vi "Create Platform Application.vi"(6 "Platform Application Attributes":T1[](array[typedef]), 7 "Region":T3, 8 "error in (no error)":errorcluster, 9 "Platform":T5, 10 "Name":string, 11 "AWS Credentials":T4) -> (0 "error out":errorcluster, 3 "Platform application out":refnum<class "Platform Application.lvclass">)   [LabVIEW 2015, in "NI_AWS_SNS.lvlib" / "Platform Application.lvclass"]
uses:
  Platform Application.lvclass
  Platform.ctl
  Core/HTTP Request/AWS Credentials.ctl
  Core/HTTP Request/Region.ctl
  Application Attribute Value Pair.ctl
  Application Attribute.ctl
  Core/HTTP Request/Name Value Pair.ctl
  Core/HTTP Request/Request Options.ctl
  Core/HTTP Request/HTTP Request.lvclass/HTTP Request.ctl
  Core/ARN/ARN.lvclass/ARN.ctl
  Core/HTTP Request/Write Credentials.vi
  Core/HTTP Request/Write Region.vi
  Core/HTTP Request/Write Service.vi
  Core/HTTP Request/Write Verify Server.vi
  Core/ARN/Write ARN.vi
  Core/HTTP Request/HTTP Request.lvclass
panel:
  out "Platform application ARN":string
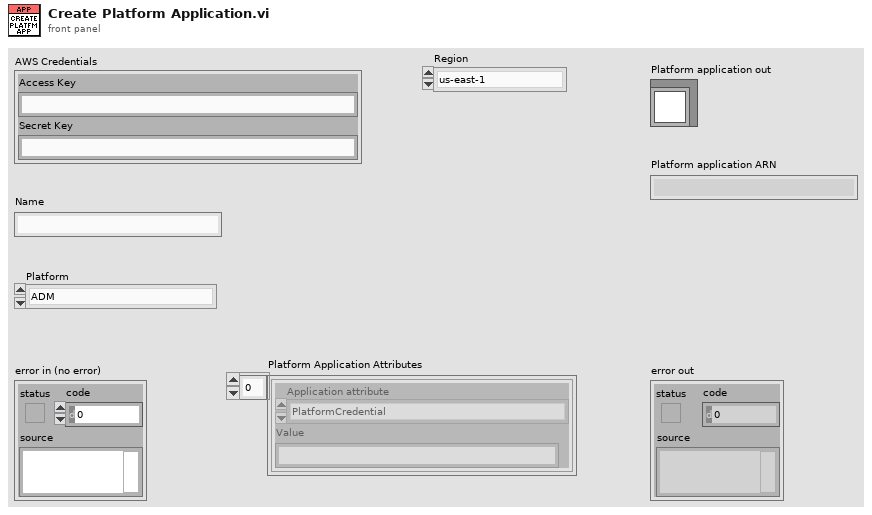
[diagram p1: front panel]
types:
  T1 = typedef "NI_AWS_SNS.lvlib/Platform Application.lvclass/Application Attribute Value Pair.ctl" = cluster{"Application attribute":T2, "Value":string}
  T2 = typedef "NI_AWS_SNS.lvlib/Platform Application.lvclass/Application Attribute.ctl" = enum16{"PlatformCredential", "PlatformPrincipal", "EventEndpointCreated", "EventEndpointDeleted", "EventEndpointUpdated", "EventDeliveryFailure", "SuccessFeedbackRoleArn", "FailureFeedbackRoleArn", "SuccessFeedbackSampleRate"}
  T3 = typedef "NI_AWS_Core.lvlib/HTTP Request.lvclass/Region.ctl" = enum16{"us-east-1", "us-east-2", "us-west-1", "us-west-2", "ap-northeast-1", "ap-northeast-2", "ap-southeast-1", "ap-southeast-2", "ca-central-1", "eu-central-1", "eu-west-1", "eu-west-2", "sa-east-1"}
  T4 = typedef "NI_AWS_Core.lvlib/HTTP Request.lvclass/AWS Credentials.ctl" = cluster{"Access Key":string, "Secret Key":string}
  T5 = typedef "NI_AWS_SNS.lvlib/Platform Application.lvclass/Platform.ctl" = enum16{"ADM", "APNS", "APNS_SANDBOX", "GCM"}
  T6 = typedef "NI_AWS_Core.lvlib/HTTP Request.lvclass/Request Options.ctl" = cluster{"request headers":T7[], "request parameters":T7[], "request body":string}
  T7 = typedef "NI_AWS_Core.lvlib/HTTP Request.lvclass/Name Value Pair.ctl" = cluster{"name":string, "value":string}
  T8 = typedef "NI_AWS_Core.lvlib/HTTP Request.lvclass/Response.ctl" = cluster{"Headers":string, "Body":string}
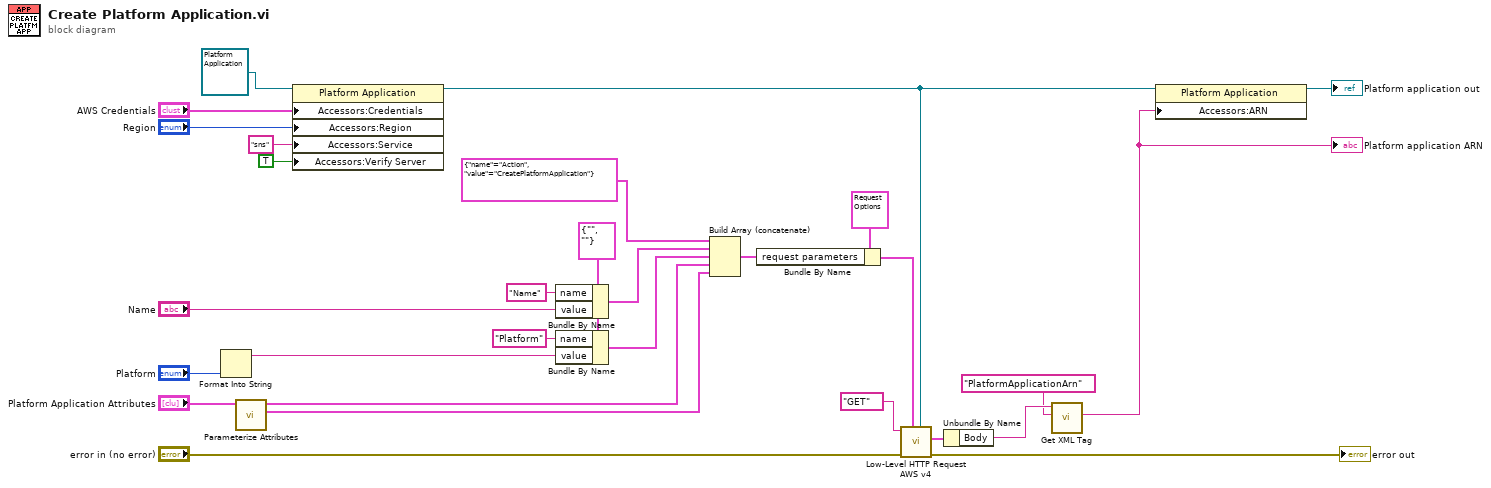
[diagram p0: block diagram]
diagram:
  w10 = T7 {"name"="", "value"=""} ("element")
  n1 = Format Into String("Platform") -> (resulting string=w7:string)  [unwired: 3 in, 1 out]
  n2 = call "Parameterize Attributes.vi"("Platform Application Attributes"="Platform Application Attributes") -> ("values"=w1:T7[], "attributes"=w2:T7[])  [unwired: 9 in]
  n3 = property class="Platform Application"(reference=refnum<class "Platform Application.lvclass"> refnum ("NI_SNS.lvclass"), "Accessors:Credentials"="AWS Credentials", "Accessors:Region"="Region", "Accessors:Service"="sns" ("Service"), "Accessors:Verify Server"=TRUE ("Verify Server")) -> (reference out=w16:refnum<class "Platform Application.lvclass">)  [unwired: 1 in, 1 out]
  n4 = Bundle By Name(cluster=w10, "name"="Name", "value"="Name") -> (w11:T7)
  n5 = Bundle By Name(cluster=w10, "name"="Platform", "value"=w7) -> (w9:T7)
  n6 = Build Array (concatenate)(T7 {"name"="Action", "value"="CreatePlatformApplication"} ("Name Value Pair"), w11, w9, w2, w1) -> (w21:T7[])
  n7 = Bundle By Name(cluster=T6 {"request headers"=[], "request parameters"=[{"name"="Action", "value"="ListQueues"}], "request body"=""} ("Request Options"), "request parameters"=w21) -> (w18:T6)
  n8 = call "Low-Level HTTP Request AWS v4.vi"("AWS Core"=w16, "Request Options"=w18, "error in (no error)"="error in (no error)", "HTTP-Verb"="GET") -> ("error out"=→"error out":errorcluster, "Response"=w17:T8)  [unwired: 5 in, 1 out]
  n9 = Unbundle By Name(w17) -> ("Body"=w6:string)
  n10 = call "Get XML Tag.vi"("Tag name"="PlatformApplicationArn" ("name"), "XML String in"=w6) -> ("Tag value"=w4:string)  [unwired: 5 in, 4 out]
  "Platform application ARN" <- w4
  n11 = property class="Platform Application"(reference=w16, "Accessors:ARN"=w4) -> (reference out=→"Platform application out":refnum<class "Platform Application.lvclass">)  [unwired: 1 in, 1 out]
